vi "List.vi"(8 "error in (no error)":errorcluster, 10 "Action":string, 11 "Policies in":refnum<class "Policies.lvclass">) -> (0 "error out":errorcluster, 2 "Roles":string[](array[string]), 3 "Policies out":refnum<class "Policies.lvclass">)   [LabVIEW 2016, in "Policies.lvclass"]
uses:
  Policies.lvclass
  Policies.lvclass/Policies.ctl
  LUT/LUT.lvclass
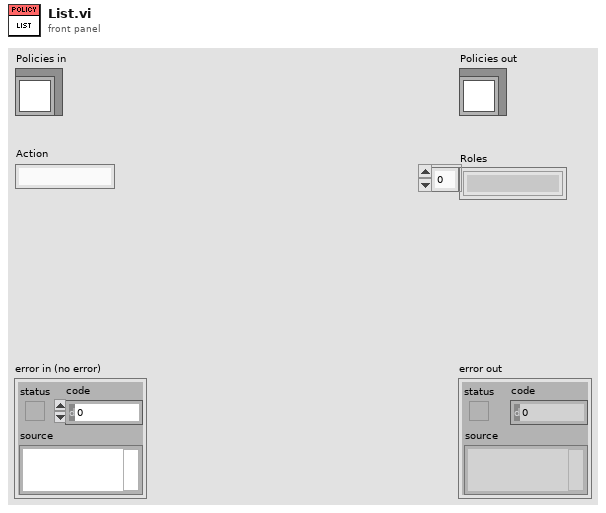
[diagram p1: front panel]
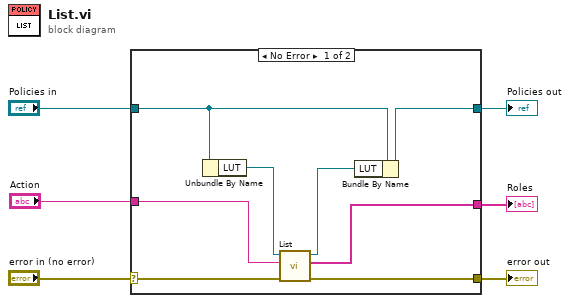
[diagram p0: block diagram]
diagram:
  n1 = case shown="No Error" "error in (no error)" {
    selector: "error in (no error)" -> [w13 w16]
    tunnel: [w12 w16] -> w5
    tunnel: [w9 w15] -> w3
    tunnel: "Policies in" -> [w14 w15]
    tunnel: "Action" -> [w10 _]
    tunnel: [w7 _] -> w1
    frame No Error {
      n2 = Unbundle By Name(w14) -> ("LUT"=w11:refnum<class "LUT.lvclass">)
      n3 = call "List.vi"("error in (no error)"=w13, "Key"=w10, "LUT in"=w11) -> ("error out"=w12:errorcluster, "Values"=w7:string[], "LUT out"=w8:refnum<class "LUT.lvclass">)  [unwired: 5 in, 1 out]
      n4 = Bundle By Name(cluster=w14, "LUT"=w8) -> (w9:refnum<class "Policies.lvclass">)
    }
    frame Error {
    }
  }
  "error out" <- w5
  "Policies out" <- w3
  "Roles" <- w1
